vi "mainActivity_初始化_需要提前开启.vi"(8 "error in (no error)":errorcluster caption="错误输入（无错误）") -> (0 "error out":errorcluster caption="错误输出")   [LabVIEW 2014]
doc: "该模板用于创建子VI。"
uses:
  R/manifest.vi
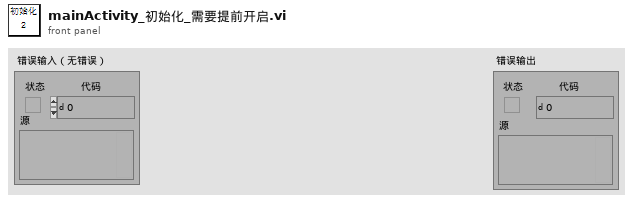
[diagram p1: front panel]
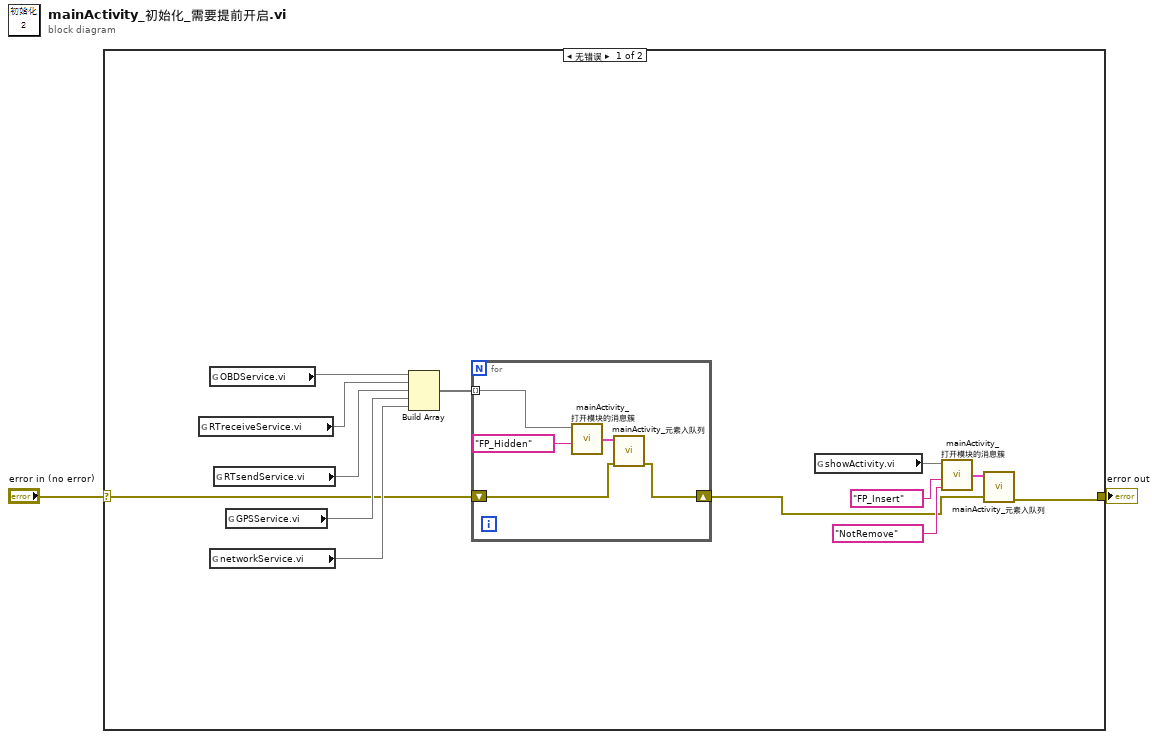
[diagram p0: block diagram]
diagram:
  n1 = case shown="无错误" "error in (no error)" {
    selector: "error in (no error)" -> [w4 w21]
    tunnel: [w11 w21] -> w1
    frame No Error {
      n2 = global read "manifest.vi" "RTreceiveService.vi"() -> (w9)
      n3 = global read "manifest.vi" "OBDService.vi"() -> (w10)
      n4 = global read "manifest.vi" "networkService.vi"() -> (w6)
      n5 = global read "manifest.vi" "RTsendService.vi"() -> (w8)
      n6 = global read "manifest.vi" "GPSService.vi"() -> (w7)
      n7 = Build Array(w10, w9, w8, w7, w6) -> (w5:void[])
      n8 = for {
        tunnel: w5 -> [w19] mode=indexing
        shift-right: [w16] -> w3
        shift-left: w4 -> [w17]
        n9 = call "mainActivity_打开模块的消息簇.vi"("前面板状态"="FP_Hidden", "模块注册信息"=w19) -> ("消息簇"=w20:cluster{"相对路径":string, string[]})  [unwired: 4 in]
        n10 = call "mainActivity_元素入队列.vi"("error in (no error)"=w17, "元素"=w20) -> ("error out"=w16:errorcluster)  [unwired: 9 in]
      }
      n11 = global read "manifest.vi" "showActivity.vi"() -> (w15)
      n12 = call "mainActivity_打开模块的消息簇.vi"("是否移除前模块"="NotRemove", "前面板状态"="FP_Insert", "模块注册信息"=w15) -> ("消息簇"=w12:cluster{"相对路径":string, string[]})  [unwired: 3 in]
      n13 = call "mainActivity_元素入队列.vi"("error in (no error)"=w3, "元素"=w12) -> ("error out"=w11:errorcluster)  [unwired: 9 in]
    }
    frame Error {
    }
  }
  "error out" <- w1
